vi "Duty Cycle Conversion.vi"(1 "Duty Cycle In":dbl(slide)=0.5 scale=-1.0..1.0) -> (0 "Duty Cyle Out":dbl)   [LabVIEW 2017]
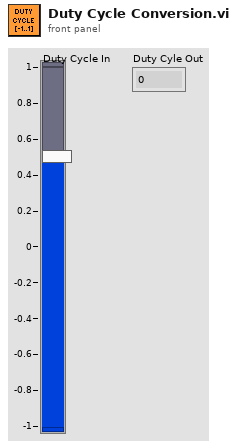
[diagram p1: front panel]
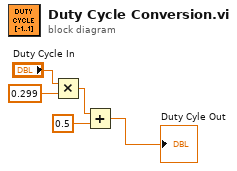
[diagram p0: block diagram]
diagram:
  n1 = Multiply(x="Duty Cycle In", y=0.299) -> (x*y=w3:dbl)
  n2 = Add(x=w3, y=0.5) -> (x+y=→"Duty Cyle Out":dbl)
